vi "Stop Logging.vi"(8 "Error In":errorcluster, 11 "Logger":refnum<class "Log.lvclass">) -> (0 "Error Out":errorcluster, 2 "sinks":refnum<class "Log Sinks.lvclass">[](array[class]))   [LabVIEW 2019, in "TSC Event Logger.lvlib" / "Log.lvclass"]
doc: "Stop the event logging actions.\n\n<b>Code Developed By:</b>\nTechnology Service Corporation\nBloomington, IN 47403\nwww.tsc.com/atcs\n\nDeveloper:\nDaniel Coons"
uses:
  Log.lvclass
  Log Sinks/Log Sinks.lvclass
  Log.lvclass/Log.ctl
  60734c66-e9c4-4f7b-8ff5-d0db667ceed0.vi
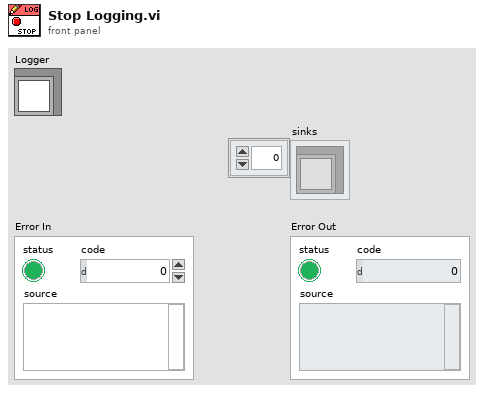
[diagram p1: front panel]
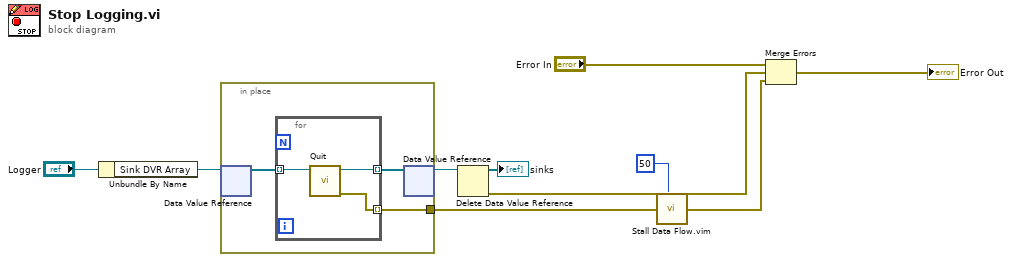
[diagram p0: block diagram]
diagram:
  n1 = Unbundle By Name("Logger") -> ("Sink DVR Array"=w6:refnum<data-value>)
  n2 = in-place {
    in-place-border: [w13] -> w9
    n3 = in-place-dvr #1(w6) -> (w12:refnum<class "Log Sinks.lvclass">[])  [unwired: 1 out]
    n4 = for {
      tunnel: [w15] -> w13 mode=indexing
      tunnel: w12 -> [w16] mode=indexing
      tunnel: [w14] -> w11 mode=indexing
      n5 = call "Quit.vi"("Log Sinks in"=w16) -> ("error out"=w15:errorcluster, "Log Sinks final"=w14:refnum<class "Log Sinks.lvclass">)  [unwired: 9 in]
    }
    n6 = in-place-dvr #1(w11) -> (w5:refnum<data-value>)  [unwired: 1 out]
  }
  n7 = Delete Data Value Reference(data value reference=w5) -> (data value=→"sinks":refnum<class "Log Sinks.lvclass">[], error out=w4:errorcluster)  [unwired: 1 in]
  n8 = call "Stall Data Flow.vim"("value in"=w9, "milliseconds to wait"=u32 50) -> ("value out"=w3:errorcluster[])  [unwired: 1 out]
  n9 = Merge Errors("Error In", w4, w3) -> (→"Error Out":errorcluster)
